vi "Return.vi"(7 "LabVIEW Web Service Request":refnum<class "Web Request.lvclass">) -> ()   [LabVIEW 2016]
uses:
  <vilib>/wsapi/Web Request.lvclass
  Device Info.ctl
  Inventory FGV Command.ctl
panel:
  out "error out":errorcluster
  # "Use the Web Service Request input terminal to call the VIs on the Web Services palette. Do not remove it from the connector pane unless you don't need access to the palette."
  # "Each additional control wired to the connector pane will be available as an input in the URL. To include an indicator in terminal-mode output (the default setting), it must also be wired to the connector pane."
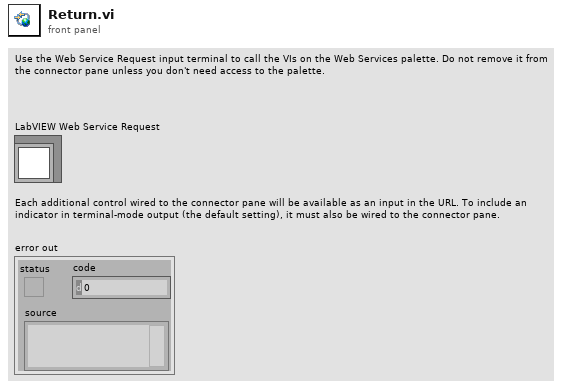
[diagram p1: front panel]
types:
  T1 = typedef "Inventory FGV Command.ctl" = enum16{"Load Items", "Check Status", "Return Items", "Check Out Items", "Add New Item", "Get All Items", "Remove Item", "Search"}
  T2 = typedef "Device Info.ctl" = cluster{"Model Number":string, "Identifier":string, "Available?":bool, "Owner":string, "Owner Email":string, "Last Activity Date":string, "Loan Purpose":string, "Department":string, "Notes":string, "Serial Number":string}
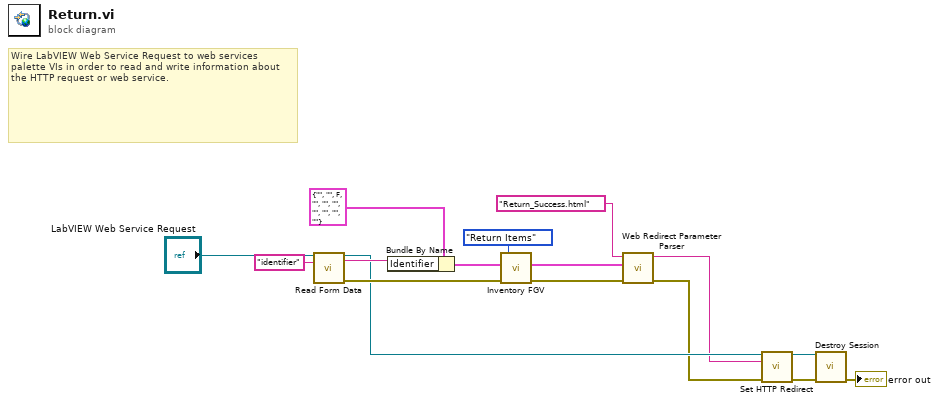
[diagram p0: block diagram]
diagram:
  # "Wire LabVIEW Web Service Request to web services palette VIs in order to read and write information about the HTTP request or web service."
  n1 = call <vilib>:"Read Form Data.vi"("LabVIEW Web Service Request"="LabVIEW Web Service Request", "key"="identifier") -> ("LabVIEW Web Service Request out"=w9:refnum<class "Web Request.lvclass">, "value"=w14:string, "error out"=w10:errorcluster)  [unwired: 10 in, 1 out]
  n2 = Bundle By Name(cluster=T2 {"Model Number"="", "Identifier"="", "Available?"=FALSE, "Owner"="", "Owner Email"="", "Last Activity Date"="", "Loan Purpose"="", "Department"="", "Notes"="", "Serial Number"=""} ("Device"), "Identifier"=w14) -> (w11:T2)
  n3 = call "Inventory FGV.vi"("error in"=w10, "Device Info"=w11, "Command"=Inventory_FGV_Command."Return Items") -> ("error out"=w5:errorcluster, "Device Info Out"=w3:T2)  [unwired: 5 in, 1 out]
  n4 = call "Web Redirect Parameter Parser.vi"("redirect URL"="Return_Success.html", "Device"=w3, "error in (no error)"=w5) -> ("Output String"=w1:string, "error out"=w2:errorcluster)  [unwired: 6 in]
  n5 = call <vilib>:"Set HTTP Redirect.vi"("LabVIEW Web Service Request"=w9, "redirect URL"=w1, "error in (no error)"=w2) -> ("LabVIEW Web Service Request out"=w8:refnum<class "Web Request.lvclass">, "error out"=w7:errorcluster)  [unwired: 11 in]
  n6 = call <vilib>:"Destroy Session.vi"("LabVIEW Web Service Request"=w8, "error in (no error)"=w7) -> ("error out"=→"error out":errorcluster)  [unwired: 12 in, 1 out]
